vi "TX.vi"() -> ()   [LabVIEW 2014]
uses:
  <vilib>/Analysis/2dsp.llb/Complex FFT.vi
  <instrlib>/niUSRP/niUSRP Fetch Rx Data (CDB).vi
  <vilib>/addons/Modulation/Digital/General/MT Map QAM Symbols to Bits.vi
  <vilib>/Analysis/NI_AALPro.lvlib
  <vilib>/addons/Modulation/niDMT.lvlib
panel:
  in  "PN sequence order (9) 2":i32=9 caption="PN sequence order (9)"
  in  "Frame Instruction 2":T1
  in  "Code Cluster":T2={"Code type"=enum."No code", "Encode factor"=2, "Constraint length(For convolution code)"=3}
  in  "modulation choice 3":T3
  in  "modulation choice 2":T3
  out "Outgoing Constellation":cdb[](graph)=[-0.7071067811865476-0.7071067811865476i, -0.7071067811865476-0.7071067811865476i, -0.7071067811865476-0.7071067811865476i, 0.7071067811865476-0.7071067811865476i, 0.7071067811865476-0.7071067811865476i, 0.7071067811865476+0.7071067811865476i, 0.7071067811865476-0.7071067811865476i, -0.7071067811865476-0.7071067811865476i, 0.7071067811865476+0.7071067811865476i, -0.7071067811865476+0.7071067811865476i, -0.7071067811865476-0.7071067811865476i, -0.7071067811865476+0.7071067811865476i, -0.7071067811865476+0.7071067811865476i, 0.7071067811865476-0.7071067811865476i, -0.7071067811865476+0.7071067811865476i, -0.7071067811865476+0.7071067811865476i, 0.7071067811865476-0.7071067811865476i, -0.7071067811865476+0.7071067811865476i, -0.7071067811865476-0.7071067811865476i, 0.7071067811865476-0.7071067811865476i, 0.7071067811865476+0.7071067811865476i, -0.7071067811865476-0.7071067811865476i, -0.7071067811865476-0.7071067811865476i, 0.7071067811865476-0.7071067811865476i, -0.7071067811865476-0.7071067811865476i, 0.7071067811865476-0.7071067811865476i, 0.7071067811865476-0.7071067811865476i, 0.7071067811865476+0.7071067811865476i, 0.7071067811865476+0.7071067811865476i, -0.7071067811865476-0.7071067811865476i, -0.7071067811865476+0.7071067811865476i, -0.7071067811865476+0.7071067811865476i, 0.7071067811865476-0.7071067811865476i, -0.7071067811865476-0.7071067811865476i, -0.7071067811865476+0.7071067811865476i, -0.7071067811865476-0.7071067811865476i, -0.7071067811865476+0.7071067811865476i, 0.7071067811865476-0.7071067811865476i, 0.7071067811865476+0.7071067811865476i, 0.7071067811865476+0.7071067811865476i, 0.7071067811865476-0.7071067811865476i, -0.7071067811865476-0.7071067811865476i, -0.7071067811865476+0.7071067811865476i, -0.7071067811865476+0.7071067811865476i, -0.7071067811865476-0.7071067811865476i, -0.7071067811865476-0.7071067811865476i, -0.7071067811865476+0.7071067811865476i, -0.7071067811865476+0.7071067811865476i, -0.7071067811865476+0.7071067811865476i, -0.7071067811865476+0.7071067811865476i, 0.7071067811865476+0.7071067811865476i, 0.7071067811865476+0.7071067811865476i, 0.7071067811865476+0.7071067811865476i, 0.7071067811865476-0.7071067811865476i, 0.7071067811865476-0.7071067811865476i, -0.7071067811865476+0.7071067811865476i, -0.7071067811865476+0.7071067811865476i, -0.7071067811865476+0.7071067811865476i, -0.7071067811865476-0.7071067811865476i, 0.7071067811865476-0.7071067811865476i, -0.7071067811865476+0.7071067811865476i, -0.7071067811865476+0.7071067811865476i, -0.7071067811865476-0.7071067811865476i, -0.7071067811865476+0.7071067811865476i, -0.7071067811865476-0.7071067811865476i, 0.7071067811865476+0.7071067811865476i, 0.7071067811865476+0.7071067811865476i, 0.7071067811865476+0.7071067811865476i, -0.7071067811865476-0.7071067811865476i, 0.7071067811865476-0.7071067811865476i, -0.7071067811865476+0.7071067811865476i, -0.7071067811865476-0.7071067811865476i, -0.7071067811865476+0.7071067811865476i, 0.7071067811865476+0.7071067811865476i, 0.7071067811865476-0.7071067811865476i, -0.7071067811865476+0.7071067811865476i, -0.7071067811865476-0.7071067811865476i, 0.7071067811865476-0.7071067811865476i, 0.7071067811865476-0.7071067811865476i, -0.7071067811865476-0.7071067811865476i, 0.7071067811865476-0.7071067811865476i, 0.7071067811865476-0.7071067811865476i, 0.7071067811865476-0.7071067811865476i, 0.7071067811865476+0.7071067811865476i, 0.7071067811865476-0.7071067811865476i, -0.7071067811865476+0.7071067811865476i, 0.7071067811865476+0.7071067811865476i, 0.7071067811865476+0.7071067811865476i, -0.7071067811865476-0.7071067811865476i, 0.7071067811865476+0.7071067811865476i, -0.7071067811865476-0.7071067811865476i, 0.7071067811865476-0.7071067811865476i, 0.7071067811865476+0.7071067811865476i, -0.7071067811865476+0.7071067811865476i, -0.7071067811865476+0.7071067811865476i, -0.7071067811865476-0.7071067811865476i, 0.7071067811865476-0.7071067811865476i, -0.7071067811865476-0.7071067811865476i, -0.7071067811865476+0.7071067811865476i, 0.7071067811865476-0.7071067811865476i, -0.7071067811865476+0.7071067811865476i, 0.7071067811865476-0.7071067811865476i, 0.7071067811865476-0.7071067811865476i, 0.7071067811865476+0.7071067811865476i, -0.7071067811865476+0.7071067811865476i, -0.7071067811865476-0.7071067811865476i, -0.7071067811865476+0.7071067811865476i, -0.7071067811865476-0.7071067811865476i, 0.7071067811865476-0.7071067811865476i, 0.7071067811865476+0.7071067811865476i, -0.7071067811865476+0.7071067811865476i, -0.7071067811865476-0.7071067811865476i, -0.7071067811865476-0.7071067811865476i, -0.7071067811865476-0.7071067811865476i, -0.7071067811865476-0.7071067811865476i, 0.7071067811865476+0.7071067811865476i, 0.7071067811865476+0.7071067811865476i, -0.7071067811865476+0.7071067811865476i, -0.7071067811865476-0.7071067811865476i, 0.7071067811865476-0.7071067811865476i, -0.7071067811865476-0.7071067811865476i, -0.7071067811865476-0.7071067811865476i, 0.7071067811865476-0.7071067811865476i, 0.7071067811865476+0.7071067811865476i, 0.7071067811865476-0.7071067811865476i, -0.7071067811865476-0.7071067811865476i, 0.7071067811865476-0.7071067811865476i, -0.7071067811865476+0.7071067811865476i, 0.7071067811865476-0.7071067811865476i, -0.7071067811865476+0.7071067811865476i, 0.7071067811865476+0.7071067811865476i, 0.7071067811865476+0.7071067811865476i, -0.7071067811865476+0.7071067811865476i, 0.7071067811865476+0.7071067811865476i, 0.7071067811865476-0.7071067811865476i, 0.7071067811865476-0.7071067811865476i, -0.7071067811865476+0.7071067811865476i, -0.7071067811865476-0.7071067811865476i, -0.7071067811865476+0.7071067811865476i, 0.7071067811865476-0.7071067811865476i, 0.7071067811865476-0.7071067811865476i, 0.7071067811865476+0.7071067811865476i, -0.7071067811865476-0.7071067811865476i, -0.7071067811865476-0.7071067811865476i, 0.7071067811865476+0.7071067811865476i, -0.7071067811865476-0.7071067811865476i, -0.7071067811865476-0.7071067811865476i, 0.7071067811865476-0.7071067811865476i, -0.7071067811865476+0.7071067811865476i, 0.7071067811865476-0.7071067811865476i, -0.7071067811865476-0.7071067811865476i, 0.7071067811865476+0.7071067811865476i, -0.7071067811865476+0.7071067811865476i, -0.7071067811865476+0.7071067811865476i, -0.7071067811865476+0.7071067811865476i, 0.7071067811865476+0.7071067811865476i, 0.7071067811865476-0.7071067811865476i, 0.7071067811865476+0.7071067811865476i, -0.7071067811865476-0.7071067811865476i, 0.7071067811865476-0.7071067811865476i, 0.7071067811865476+0.7071067811865476i, -0.7071067811865476-0.7071067811865476i, -0.7071067811865476+0.7071067811865476i, 0.7071067811865476-0.7071067811865476i, 0.7071067811865476-0.7071067811865476i, 0.7071067811865476-0.7071067811865476i, -0.7071067811865476-0.7071067811865476i, 0.7071067811865476-0.7071067811865476i, 0.7071067811865476+0.7071067811865476i, 0.7071067811865476-0.7071067811865476i, -0.7071067811865476+0.7071067811865476i, 0.7071067811865476-0.7071067811865476i, 0.7071067811865476+0.7071067811865476i, 0.7071067811865476-0.7071067811865476i, 0.7071067811865476+0.7071067811865476i, 0.7071067811865476-0.7071067811865476i, 0.7071067811865476+0.7071067811865476i, 0.7071067811865476+0.7071067811865476i, 0.7071067811865476+0.7071067811865476i, -0.7071067811865476+0.7071067811865476i, 0.7071067811865476+0.7071067811865476i, 0.7071067811865476+0.7071067811865476i, 0.7071067811865476-0.7071067811865476i, 0.7071067811865476+0.7071067811865476i, -0.7071067811865476-0.7071067811865476i, 0.7071067811865476+0.7071067811865476i, 0.7071067811865476+0.7071067811865476i, 0.7071067811865476-0.7071067811865476i, -0.7071067811865476+0.7071067811865476i, -0.7071067811865476-0.7071067811865476i, 0.7071067811865476+0.7071067811865476i, 0.7071067811865476-0.7071067811865476i, 0.7071067811865476-0.7071067811865476i, 0.7071067811865476-0.7071067811865476i, -0.7071067811865476-0.7071067811865476i, 0.7071067811865476+0.7071067811865476i, 0.7071067811865476+0.7071067811865476i, -0.7071067811865476-0.7071067811865476i, -0.7071067811865476+0.7071067811865476i, -0.7071067811865476-0.7071067811865476i, 0.7071067811865476-0.7071067811865476i, 0.7071067811865476-0.7071067811865476i, -0.7071067811865476+0.7071067811865476i, 0.7071067811865476-0.7071067811865476i, -0.7071067811865476-0.7071067811865476i, 0.7071067811865476-0.7071067811865476i, -0.7071067811865476+0.7071067811865476i, 0.7071067811865476+0.7071067811865476i, -0.7071067811865476+0.7071067811865476i, -0.7071067811865476+0.7071067811865476i, 0.7071067811865476+0.7071067811865476i, 0.7071067811865476+0.7071067811865476i, 0.7071067811865476-0.7071067811865476i, 0.7071067811865476-0.7071067811865476i, -0.7071067811865476-0.7071067811865476i, -0.7071067811865476+0.7071067811865476i, 0.7071067811865476+0.7071067811865476i, -0.7071067811865476-0.7071067811865476i, -0.7071067811865476-0.7071067811865476i, -0.7071067811865476-0.7071067811865476i, -0.7071067811865476+0.7071067811865476i, 0.7071067811865476-0.7071067811865476i, -0.7071067811865476+0.7071067811865476i, 0.7071067811865476+0.7071067811865476i, 0.7071067811865476-0.7071067811865476i, -0.7071067811865476+0.7071067811865476i, -0.7071067811865476+0.7071067811865476i, 0.7071067811865476-0.7071067811865476i, -0.7071067811865476-0.7071067811865476i, -0.7071067811865476-0.7071067811865476i, -0.7071067811865476-0.7071067811865476i, 0.7071067811865476+0.7071067811865476i, 0.7071067811865476-0.7071067811865476i, -0.7071067811865476+0.7071067811865476i, 0.7071067811865476-0.7071067811865476i, 0.7071067811865476-0.7071067811865476i, 0.7071067811865476-0.7071067811865476i, -0.7071067811865476+0.7071067811865476i, 0.7071067811865476-0.7071067811865476i, -0.7071067811865476+0.7071067811865476i, 0.7071067811865476-0.7071067811865476i, 0.7071067811865476+0.7071067811865476i, 0.7071067811865476+0.7071067811865476i, 0.7071067811865476+0.7071067811865476i, -0.7071067811865476-0.7071067811865476i, 0.7071067811865476+0.7071067811865476i, -0.7071067811865476+0.7071067811865476i, 0.7071067811865476-0.7071067811865476i, -0.7071067811865476+0.7071067811865476i, -0.7071067811865476+0.7071067811865476i, 0.7071067811865476+0.7071067811865476i, -0.7071067811865476+0.7071067811865476i, 0.7071067811865476-0.7071067811865476i, 0.7071067811865476-0.7071067811865476i, -0.7071067811865476+0.7071067811865476i, -0.7071067811865476+0.7071067811865476i, -0.7071067811865476-0.7071067811865476i, -0.7071067811865476-0.7071067811865476i, -0.7071067811865476-0.7071067811865476i, -0.7071067811865476+0.7071067811865476i, 0.7071067811865476+0.7071067811865476i, -0.7071067811865476+0.7071067811865476i, -0.7071067811865476+0.7071067811865476i, 0.7071067811865476-0.7071067811865476i, 0.7071067811865476+0.7071067811865476i, -0.7071067811865476-0.7071067811865476i, 0.7071067811865476-0.7071067811865476i, 0.7071067811865476-0.7071067811865476i, -0.7071067811865476-0.7071067811865476i, 0.7071067811865476+0.7071067811865476i, 0.7071067811865476-0.7071067811865476i, -0.7071067811865476-0.7071067811865476i, 0.7071067811865476+0.7071067811865476i, -0.7071067811865476-0.7071067811865476i, -0.7071067811865476-0.7071067811865476i, 0.7071067811865476+0.7071067811865476i, -0.7071067811865476+0.7071067811865476i, -0.7071067811865476-0.7071067811865476i, -0.7071067811865476-0.7071067811865476i, -0.7071067811865476+0.7071067811865476i, -0.7071067811865476-0.7071067811865476i, -0.7071067811865476+0.7071067811865476i, 0.7071067811865476+0.7071067811865476i, 0.7071067811865476+0.7071067811865476i, -0.7071067811865476+0.7071067811865476i, 0.7071067811865476-0.7071067811865476i, 0.7071067811865476-0.7071067811865476i, -0.7071067811865476-0.7071067811865476i, -0.7071067811865476+0.7071067811865476i, 0.7071067811865476-0.7071067811865476i, -0.7071067811865476-0.7071067811865476i, 0.7071067811865476-0.7071067811865476i, -0.7071067811865476-0.7071067811865476i, 0.7071067811865476+0.7071067811865476i, 0.7071067811865476+0.7071067811865476i, -0.7071067811865476+0.7071067811865476i, -0.7071067811865476+0.7071067811865476i, 0.7071067811865476-0.7071067811865476i, 0.7071067811865476-0.7071067811865476i, -0.7071067811865476-0.7071067811865476i, -0.7071067811865476-0.7071067811865476i, 0.7071067811865476-0.7071067811865476i, 0.7071067811865476-0.7071067811865476i, 0.7071067811865476-0.7071067811865476i, 0.7071067811865476-0.7071067811865476i, 0.7071067811865476-0.7071067811865476i, 0.7071067811865476+0.7071067811865476i, 0.7071067811865476+0.7071067811865476i, -0.7071067811865476+0.7071067811865476i, -0.7071067811865476+0.7071067811865476i, 0.7071067811865476+0.7071067811865476i, 0.7071067811865476-0.7071067811865476i, 0.7071067811865476-0.7071067811865476i, -0.7071067811865476-0.7071067811865476i, -0.7071067811865476-0.7071067811865476i, 0.7071067811865476+0.7071067811865476i, 0.7071067811865476-0.7071067811865476i, -0.7071067811865476-0.7071067811865476i, 0.7071067811865476-0.7071067811865476i, -0.7071067811865476-0.7071067811865476i, 0.7071067811865476-0.7071067811865476i, 0.7071067811865476+0.7071067811865476i, 0.7071067811865476+0.7071067811865476i, -0.7071067811865476+0.7071067811865476i, -0.7071067811865476-0.7071067811865476i, 0.7071067811865476+0.7071067811865476i, -0.7071067811865476-0.7071067811865476i, 0.7071067811865476-0.7071067811865476i, 0.7071067811865476-0.7071067811865476i, -0.7071067811865476+0.7071067811865476i, 0.7071067811865476+0.7071067811865476i, -0.7071067811865476-0.7071067811865476i, -0.7071067811865476-0.7071067811865476i, -0.7071067811865476+0.7071067811865476i, -0.7071067811865476+0.7071067811865476i, -0.7071067811865476-0.7071067811865476i, -0.7071067811865476+0.7071067811865476i, -0.7071067811865476+0.7071067811865476i, 0.7071067811865476+0.7071067811865476i, -0.7071067811865476+0.7071067811865476i, 0.7071067811865476+0.7071067811865476i, 0.7071067811865476-0.7071067811865476i, 0.7071067811865476+0.7071067811865476i, -0.7071067811865476+0.7071067811865476i, 0.7071067811865476-0.7071067811865476i, -0.7071067811865476+0.7071067811865476i, -0.7071067811865476-0.7071067811865476i, 0.7071067811865476+0.7071067811865476i, 0.7071067811865476+0.7071067811865476i, 0.7071067811865476-0.7071067811865476i, -0.7071067811865476-0.7071067811865476i, -0.7071067811865476-0.7071067811865476i, -0.7071067811865476+0.7071067811865476i, 0.7071067811865476-0.7071067811865476i, -0.7071067811865476-0.7071067811865476i, 0.7071067811865476+0.7071067811865476i, -0.7071067811865476-0.7071067811865476i, -0.7071067811865476+0.7071067811865476i, 0.7071067811865476+0.7071067811865476i, 0.7071067811865476+0.7071067811865476i, -0.7071067811865476-0.7071067811865476i, 0.7071067811865476-0.7071067811865476i, -0.7071067811865476-0.7071067811865476i, -0.7071067811865476-0.7071067811865476i, 0.7071067811865476+0.7071067811865476i, 0.7071067811865476+0.7071067811865476i, -0.7071067811865476-0.7071067811865476i, -0.7071067811865476-0.7071067811865476i, -0.7071067811865476-0.7071067811865476i, -0.7071067811865476-0.7071067811865476i, 0.7071067811865476-0.7071067811865476i, 0.7071067811865476+0.7071067811865476i, 0.7071067811865476+0.7071067811865476i, -0.7071067811865476-0.7071067811865476i, -0.7071067811865476-0.7071067811865476i, -0.7071067811865476+0.7071067811865476i, -0.7071067811865476-0.7071067811865476i, -0.7071067811865476-0.7071067811865476i, 0.7071067811865476+0.7071067811865476i, -0.7071067811865476+0.7071067811865476i, -0.7071067811865476+0.7071067811865476i, -0.7071067811865476-0.7071067811865476i, 0.7071067811865476+0.7071067811865476i, -0.7071067811865476-0.7071067811865476i, 0.7071067811865476+0.7071067811865476i, 0.7071067811865476-0.7071067811865476i, 0.7071067811865476+0.7071067811865476i, 0.7071067811865476+0.7071067811865476i, 0.7071067811865476-0.7071067811865476i, -0.7071067811865476+0.7071067811865476i, -0.7071067811865476+0.7071067811865476i, 0.7071067811865476+0.7071067811865476i, -0.7071067811865476-0.7071067811865476i, 0.7071067811865476-0.7071067811865476i, -0.7071067811865476-0.7071067811865476i, -0.7071067811865476+0.7071067811865476i, 0.7071067811865476+0.7071067811865476i, -0.7071067811865476+0.7071067811865476i, -0.7071067811865476-0.7071067811865476i, 0.7071067811865476-0.7071067811865476i, -0.7071067811865476+0.7071067811865476i, -0.7071067811865476-0.7071067811865476i, -0.7071067811865476-0.7071067811865476i, 0.7071067811865476+0.7071067811865476i, -0.7071067811865476-0.7071067811865476i, -0.7071067811865476+0.7071067811865476i, 0.7071067811865476-0.7071067811865476i, 0.7071067811865476+0.7071067811865476i, 0.7071067811865476-0.7071067811865476i, 0.7071067811865476-0.7071067811865476i, 0.7071067811865476-0.7071067811865476i, -0.7071067811865476+0.7071067811865476i, 0.7071067811865476+0.7071067811865476i, -0.7071067811865476+0.7071067811865476i, -0.7071067811865476-0.7071067811865476i, 0.7071067811865476+0.7071067811865476i, -0.7071067811865476+0.7071067811865476i, 0.7071067811865476-0.7071067811865476i, -0.7071067811865476-0.7071067811865476i, -0.7071067811865476+0.7071067811865476i, -0.7071067811865476+0.7071067811865476i, -0.7071067811865476+0.7071067811865476i, -0.7071067811865476-0.7071067811865476i, 0.7071067811865476+0.7071067811865476i, -0.7071067811865476+0.7071067811865476i, 0.7071067811865476+0.7071067811865476i, -0.7071067811865476-0.7071067811865476i, 0.7071067811865476+0.7071067811865476i, -0.7071067811865476+0.7071067811865476i, 0.7071067811865476+0.7071067811865476i, -0.7071067811865476+0.7071067811865476i, 0.7071067811865476+0.7071067811865476i, 0.7071067811865476+0.7071067811865476i, 0.7071067811865476+0.7071067811865476i, 0.7071067811865476+0.7071067811865476i, 0.7071067811865476-0.7071067811865476i, 0.7071067811865476+0.7071067811865476i, -0.7071067811865476+0.7071067811865476i, 0.7071067811865476+0.7071067811865476i, -0.7071067811865476+0.7071067811865476i, 0.7071067811865476-0.7071067811865476i, 0.7071067811865476+0.7071067811865476i, -0.7071067811865476+0.7071067811865476i, 0.7071067811865476+0.7071067811865476i, -0.7071067811865476-0.7071067811865476i, 0.7071067811865476-0.7071067811865476i, -0.7071067811865476+0.7071067811865476i, -0.7071067811865476+0.7071067811865476i, -0.7071067811865476+0.7071067811865476i, -0.7071067811865476+0.7071067811865476i, 0.7071067811865476-0.7071067811865476i, 0.7071067811865476+0.7071067811865476i, -0.7071067811865476+0.7071067811865476i, 0.7071067811865476-0.7071067811865476i, -0.7071067811865476-0.7071067811865476i, -0.7071067811865476-0.7071067811865476i, -0.7071067811865476+0.7071067811865476i, 0.7071067811865476+0.7071067811865476i, -0.7071067811865476-0.7071067811865476i, -0.7071067811865476+0.7071067811865476i, -0.7071067811865476-0.7071067811865476i, 0.7071067811865476+0.7071067811865476i, 0.7071067811865476-0.7071067811865476i, 0.7071067811865476+0.7071067811865476i, 0.7071067811865476-0.7071067811865476i, 0.7071067811865476-0.7071067811865476i, 0.7071067811865476+0.7071067811865476i, -0.7071067811865476+0.7071067811865476i, -0.7071067811865476+0.7071067811865476i, -0.7071067811865476+0.7071067811865476i, 0.7071067811865476-0.7071067811865476i, 0.7071067811865476-0.7071067811865476i, -0.7071067811865476+0.7071067811865476i, -0.7071067811865476-0.7071067811865476i, -0.7071067811865476-0.7071067811865476i, 0.7071067811865476-0.7071067811865476i, -0.7071067811865476-0.7071067811865476i, 0.7071067811865476+0.7071067811865476i, 0.7071067811865476-0.7071067811865476i, -0.7071067811865476+0.7071067811865476i, 0.7071067811865476+0.7071067811865476i, 0.7071067811865476-0.7071067811865476i, -0.7071067811865476-0.7071067811865476i, -0.7071067811865476+0.7071067811865476i, -0.7071067811865476-0.7071067811865476i, -0.7071067811865476-0.7071067811865476i, 0.7071067811865476-0.7071067811865476i, -0.7071067811865476+0.7071067811865476i, 0.7071067811865476+0.7071067811865476i, -0.7071067811865476-0.7071067811865476i, -0.7071067811865476+0.7071067811865476i, -0.7071067811865476+0.7071067811865476i, 0.7071067811865476+0.7071067811865476i, -0.7071067811865476-0.7071067811865476i, 0.7071067811865476+0.7071067811865476i, -0.7071067811865476-0.7071067811865476i, 0.7071067811865476+0.7071067811865476i, 0.7071067811865476+0.7071067811865476i, 0.7071067811865476+0.7071067811865476i, -0.7071067811865476+0.7071067811865476i, 0.7071067811865476-0.7071067811865476i, 0.7071067811865476+0.7071067811865476i, -0.7071067811865476-0.7071067811865476i, 0.7071067811865476+0.7071067811865476i, 0.7071067811865476-0.7071067811865476i, 0.7071067811865476-0.7071067811865476i, 0.7071067811865476+0.7071067811865476i, -0.7071067811865476-0.7071067811865476i, -0.7071067811865476+0.7071067811865476i, 0.7071067811865476+0.7071067811865476i, 0.7071067811865476-0.7071067811865476i, -0.7071067811865476-0.7071067811865476i, -0.7071067811865476-0.7071067811865476i, -0.7071067811865476-0.7071067811865476i, 0.7071067811865476-0.7071067811865476i, 0.7071067811865476-0.7071067811865476i, 0.7071067811865476+0.7071067811865476i, 0.7071067811865476-0.7071067811865476i, -0.7071067811865476-0.7071067811865476i, 0.7071067811865476+0.7071067811865476i, -0.7071067811865476+0.7071067811865476i, -0.7071067811865476-0.7071067811865476i, -0.7071067811865476+0.7071067811865476i, -0.7071067811865476+0.7071067811865476i, 0.7071067811865476-0.7071067811865476i, -0.7071067811865476+0.7071067811865476i, -0.7071067811865476+0.7071067811865476i, 0.7071067811865476-0.7071067811865476i, -0.7071067811865476+0.7071067811865476i, -0.7071067811865476-0.7071067811865476i, 0.7071067811865476-0.7071067811865476i, 0.7071067811865476+0.7071067811865476i, -0.7071067811865476-0.7071067811865476i, -0.7071067811865476-0.7071067811865476i, 0.7071067811865476-0.7071067811865476i, -0.7071067811865476-0.7071067811865476i, 0.7071067811865476-0.7071067811865476i, 0.7071067811865476-0.7071067811865476i, 0.7071067811865476+0.7071067811865476i, 0.7071067811865476+0.7071067811865476i, -0.7071067811865476-0.7071067811865476i, -0.7071067811865476+0.7071067811865476i, -0.7071067811865476+0.7071067811865476i, 0.7071067811865476-0.7071067811865476i, -0.7071067811865476-0.7071067811865476i, -0.7071067811865476+0.7071067811865476i, -0.7071067811865476-0.7071067811865476i, -0.7071067811865476+0.7071067811865476i, 0.7071067811865476-0.7071067811865476i, 0.7071067811865476+0.7071067811865476i, 0.7071067811865476+0.7071067811865476i, 0.7071067811865476-0.7071067811865476i, -0.7071067811865476-0.7071067811865476i, -0.7071067811865476+0.7071067811865476i, -0.7071067811865476+0.7071067811865476i, -0.7071067811865476-0.7071067811865476i, -0.7071067811865476-0.7071067811865476i, -0.7071067811865476+0.7071067811865476i, -0.7071067811865476+0.7071067811865476i, -0.7071067811865476+0.7071067811865476i, -0.7071067811865476+0.7071067811865476i, 0.7071067811865476+0.7071067811865476i, 0.7071067811865476+0.7071067811865476i, 0.7071067811865476+0.7071067811865476i, 0.7071067811865476-0.7071067811865476i, 0.7071067811865476-0.7071067811865476i, -0.7071067811865476+0.7071067811865476i, -0.7071067811865476+0.7071067811865476i, -0.7071067811865476+0.7071067811865476i, -0.7071067811865476-0.7071067811865476i, 0.7071067811865476-0.7071067811865476i, -0.7071067811865476+0.7071067811865476i, -0.7071067811865476+0.7071067811865476i, -0.7071067811865476-0.7071067811865476i, -0.7071067811865476+0.7071067811865476i, -0.7071067811865476-0.7071067811865476i, 0.7071067811865476+0.7071067811865476i, 0.7071067811865476+0.7071067811865476i, 0.7071067811865476+0.7071067811865476i, -0.7071067811865476-0.7071067811865476i, 0.7071067811865476-0.7071067811865476i, -0.7071067811865476+0.7071067811865476i, -0.7071067811865476-0.7071067811865476i, -0.7071067811865476+0.7071067811865476i, 0.7071067811865476+0.7071067811865476i, 0.7071067811865476-0.7071067811865476i, -0.7071067811865476+0.7071067811865476i, -0.7071067811865476-0.7071067811865476i, 0.7071067811865476-0.7071067811865476i, 0.7071067811865476-0.7071067811865476i, -0.7071067811865476-0.7071067811865476i, 0.7071067811865476-0.7071067811865476i, 0.7071067811865476-0.7071067811865476i, 0.7071067811865476-0.7071067811865476i, 0.7071067811865476+0.7071067811865476i, 0.7071067811865476-0.7071067811865476i, -0.7071067811865476+0.7071067811865476i, 0.7071067811865476+0.7071067811865476i, 0.7071067811865476+0.7071067811865476i, -0.7071067811865476-0.7071067811865476i, 0.7071067811865476+0.7071067811865476i, -0.7071067811865476-0.7071067811865476i, 0.7071067811865476-0.7071067811865476i, 0.7071067811865476+0.7071067811865476i, -0.7071067811865476+0.7071067811865476i, -0.7071067811865476+0.7071067811865476i, -0.7071067811865476-0.7071067811865476i, 0.7071067811865476-0.7071067811865476i, -0.7071067811865476-0.7071067811865476i, -0.7071067811865476+0.7071067811865476i, 0.7071067811865476-0.7071067811865476i, -0.7071067811865476+0.7071067811865476i, 0.7071067811865476-0.7071067811865476i, 0.7071067811865476-0.7071067811865476i, 0.7071067811865476+0.7071067811865476i, -0.7071067811865476+0.7071067811865476i, -0.7071067811865476-0.7071067811865476i, -0.7071067811865476+0.7071067811865476i, -0.7071067811865476-0.7071067811865476i, 0.7071067811865476-0.7071067811865476i, 0.7071067811865476+0.7071067811865476i, -0.7071067811865476+0.7071067811865476i, -0.7071067811865476-0.7071067811865476i, -0.7071067811865476-0.7071067811865476i, -0.7071067811865476-0.7071067811865476i, -0.7071067811865476-0.7071067811865476i, 0.7071067811865476+0.7071067811865476i, 0.7071067811865476+0.7071067811865476i, -0.7071067811865476+0.7071067811865476i, -0.7071067811865476-0.7071067811865476i, 0.7071067811865476-0.7071067811865476i, -0.7071067811865476-0.7071067811865476i, -0.7071067811865476-0.7071067811865476i, 0.7071067811865476-0.7071067811865476i, 0.7071067811865476+0.7071067811865476i, 0.7071067811865476-0.7071067811865476i, -0.7071067811865476-0.7071067811865476i, 0.7071067811865476-0.7071067811865476i, -0.7071067811865476+0.7071067811865476i, 0.7071067811865476-0.7071067811865476i, -0.7071067811865476+0.7071067811865476i, 0.7071067811865476+0.7071067811865476i, 0.7071067811865476+0.7071067811865476i, -0.7071067811865476+0.7071067811865476i, 0.7071067811865476+0.7071067811865476i, 0.7071067811865476-0.7071067811865476i, 0.7071067811865476-0.7071067811865476i, -0.7071067811865476+0.7071067811865476i, -0.7071067811865476-0.7071067811865476i, -0.7071067811865476+0.7071067811865476i, 0.7071067811865476-0.7071067811865476i, 0.7071067811865476-0.7071067811865476i, 0.7071067811865476+0.7071067811865476i, -0.7071067811865476-0.7071067811865476i, -0.7071067811865476-0.7071067811865476i, 0.7071067811865476+0.7071067811865476i, -0.7071067811865476-0.7071067811865476i, -0.7071067811865476-0.7071067811865476i, 0.7071067811865476-0.7071067811865476i, -0.7071067811865476+0.7071067811865476i, 0.7071067811865476-0.7071067811865476i, -0.7071067811865476-0.7071067811865476i, 0.7071067811865476+0.7071067811865476i, -0.7071067811865476+0.7071067811865476i, -0.7071067811865476+0.7071067811865476i, -0.7071067811865476+0.7071067811865476i, 0.7071067811865476+0.7071067811865476i, 0.7071067811865476-0.7071067811865476i, 0.7071067811865476+0.7071067811865476i, -0.7071067811865476-0.7071067811865476i, 0.7071067811865476-0.7071067811865476i, 0.7071067811865476+0.7071067811865476i, -0.7071067811865476-0.7071067811865476i, -0.7071067811865476+0.7071067811865476i, 0.7071067811865476-0.7071067811865476i, 0.7071067811865476-0.7071067811865476i, 0.7071067811865476-0.7071067811865476i, -0.7071067811865476-0.7071067811865476i, 0.7071067811865476-0.7071067811865476i, 0.7071067811865476+0.7071067811865476i, 0.7071067811865476-0.7071067811865476i, -0.7071067811865476+0.7071067811865476i, 0.7071067811865476-0.7071067811865476i, 0.7071067811865476+0.7071067811865476i, 0.7071067811865476-0.7071067811865476i, 0.7071067811865476+0.7071067811865476i, 0.7071067811865476-0.7071067811865476i, 0.7071067811865476+0.7071067811865476i, 0.7071067811865476+0.7071067811865476i, 0.7071067811865476+0.7071067811865476i, -0.7071067811865476+0.7071067811865476i, 0.7071067811865476+0.7071067811865476i, 0.7071067811865476+0.7071067811865476i, 0.7071067811865476-0.7071067811865476i, 0.7071067811865476+0.7071067811865476i, -0.7071067811865476-0.7071067811865476i, 0.7071067811865476+0.7071067811865476i, 0.7071067811865476+0.7071067811865476i, 0.7071067811865476-0.7071067811865476i, -0.7071067811865476+0.7071067811865476i, -0.7071067811865476-0.7071067811865476i, 0.7071067811865476+0.7071067811865476i, 0.7071067811865476-0.7071067811865476i, 0.7071067811865476-0.7071067811865476i, 0.7071067811865476-0.7071067811865476i, -0.7071067811865476-0.7071067811865476i, 0.7071067811865476+0.7071067811865476i, 0.7071067811865476+0.7071067811865476i, -0.7071067811865476-0.7071067811865476i, -0.7071067811865476+0.7071067811865476i, -0.7071067811865476-0.7071067811865476i, 0.7071067811865476-0.7071067811865476i, 0.7071067811865476-0.7071067811865476i, -0.7071067811865476+0.7071067811865476i, 0.7071067811865476-0.7071067811865476i, -0.7071067811865476-0.7071067811865476i, 0.7071067811865476-0.7071067811865476i, -0.7071067811865476+0.7071067811865476i, 0.7071067811865476+0.7071067811865476i, -0.7071067811865476+0.7071067811865476i, -0.7071067811865476+0.7071067811865476i, 0.7071067811865476+0.7071067811865476i, 0.7071067811865476+0.7071067811865476i, 0.7071067811865476-0.7071067811865476i, 0.7071067811865476-0.7071067811865476i, -0.7071067811865476-0.7071067811865476i, -0.7071067811865476+0.7071067811865476i, 0.7071067811865476+0.7071067811865476i, -0.7071067811865476-0.7071067811865476i, -0.7071067811865476-0.7071067811865476i, -0.7071067811865476-0.7071067811865476i, -0.7071067811865476+0.7071067811865476i, 0.7071067811865476-0.7071067811865476i, -0.7071067811865476+0.7071067811865476i, 0.7071067811865476+0.7071067811865476i, 0.7071067811865476-0.7071067811865476i, -0.7071067811865476+0.7071067811865476i, -0.7071067811865476+0.7071067811865476i, 0.7071067811865476-0.7071067811865476i, -0.7071067811865476-0.7071067811865476i, -0.7071067811865476-0.7071067811865476i, -0.7071067811865476-0.7071067811865476i, 0.7071067811865476+0.7071067811865476i, 0.7071067811865476-0.7071067811865476i, -0.7071067811865476+0.7071067811865476i, 0.7071067811865476-0.7071067811865476i, 0.7071067811865476-0.7071067811865476i, 0.7071067811865476-0.7071067811865476i, -0.7071067811865476+0.7071067811865476i, 0.7071067811865476-0.7071067811865476i, -0.7071067811865476+0.7071067811865476i, 0.7071067811865476-0.7071067811865476i, 0.7071067811865476+0.7071067811865476i, 0.7071067811865476+0.7071067811865476i, 0.7071067811865476+0.7071067811865476i, -0.7071067811865476-0.7071067811865476i, 0.7071067811865476+0.7071067811865476i, -0.7071067811865476+0.7071067811865476i, 0.7071067811865476-0.7071067811865476i, -0.7071067811865476+0.7071067811865476i, -0.7071067811865476+0.7071067811865476i, 0.7071067811865476+0.7071067811865476i, -0.7071067811865476+0.7071067811865476i, 0.7071067811865476-0.7071067811865476i, 0.7071067811865476-0.7071067811865476i, -0.7071067811865476+0.7071067811865476i, -0.7071067811865476+0.7071067811865476i, -0.7071067811865476-0.7071067811865476i, -0.7071067811865476-0.7071067811865476i, -0.7071067811865476-0.7071067811865476i, -0.7071067811865476+0.7071067811865476i, 0.7071067811865476+0.7071067811865476i, -0.7071067811865476+0.7071067811865476i, -0.7071067811865476+0.7071067811865476i, 0.7071067811865476-0.7071067811865476i, 0.7071067811865476+0.7071067811865476i, -0.7071067811865476-0.7071067811865476i, 0.7071067811865476-0.7071067811865476i, 0.7071067811865476-0.7071067811865476i, -0.7071067811865476-0.7071067811865476i, 0.7071067811865476+0.7071067811865476i, 0.7071067811865476-0.7071067811865476i, -0.7071067811865476-0.7071067811865476i, 0.7071067811865476+0.7071067811865476i, -0.7071067811865476-0.7071067811865476i, -0.7071067811865476-0.7071067811865476i, 0.7071067811865476+0.7071067811865476i, -0.7071067811865476+0.7071067811865476i, -0.7071067811865476-0.7071067811865476i, -0.7071067811865476-0.7071067811865476i, -0.7071067811865476+0.7071067811865476i, -0.7071067811865476-0.7071067811865476i, -0.7071067811865476+0.7071067811865476i, 0.7071067811865476+0.7071067811865476i, 0.7071067811865476+0.7071067811865476i, -0.7071067811865476+0.7071067811865476i, 0.7071067811865476-0.7071067811865476i, 0.7071067811865476-0.7071067811865476i, -0.7071067811865476-0.7071067811865476i, -0.7071067811865476+0.7071067811865476i, 0.7071067811865476-0.7071067811865476i, -0.7071067811865476-0.7071067811865476i, 0.7071067811865476-0.7071067811865476i, -0.7071067811865476-0.7071067811865476i, 0.7071067811865476+0.7071067811865476i, 0.7071067811865476+0.7071067811865476i, -0.7071067811865476+0.7071067811865476i, -0.7071067811865476+0.7071067811865476i, 0.7071067811865476-0.7071067811865476i, 0.7071067811865476-0.7071067811865476i, -0.7071067811865476-0.7071067811865476i, -0.7071067811865476-0.7071067811865476i, 0.7071067811865476-0.7071067811865476i, 0.7071067811865476-0.7071067811865476i, 0.7071067811865476-0.7071067811865476i, 0.7071067811865476-0.7071067811865476i, 0.7071067811865476-0.7071067811865476i, 0.7071067811865476+0.7071067811865476i, 0.7071067811865476+0.7071067811865476i, -0.7071067811865476+0.7071067811865476i, -0.7071067811865476+0.7071067811865476i, 0.7071067811865476+0.7071067811865476i, 0.7071067811865476-0.7071067811865476i, 0.7071067811865476-0.7071067811865476i, -0.7071067811865476-0.7071067811865476i, -0.7071067811865476-0.7071067811865476i, 0.7071067811865476+0.7071067811865476i, 0.7071067811865476-0.7071067811865476i, -0.7071067811865476-0.7071067811865476i, 0.7071067811865476-0.7071067811865476i, -0.7071067811865476-0.7071067811865476i, 0.7071067811865476-0.7071067811865476i, 0.7071067811865476+0.7071067811865476i, 0.7071067811865476+0.7071067811865476i, -0.7071067811865476+0.7071067811865476i, -0.7071067811865476-0.7071067811865476i, 0.7071067811865476+0.7071067811865476i, -0.7071067811865476-0.7071067811865476i, 0.7071067811865476-0.7071067811865476i, 0.7071067811865476-0.7071067811865476i, -0.7071067811865476+0.7071067811865476i, 0.7071067811865476+0.7071067811865476i, -0.7071067811865476-0.7071067811865476i, -0.7071067811865476-0.7071067811865476i, -0.7071067811865476+0.7071067811865476i, -0.7071067811865476+0.7071067811865476i, -0.7071067811865476-0.7071067811865476i, -0.7071067811865476+0.7071067811865476i, -0.7071067811865476+0.7071067811865476i, 0.7071067811865476+0.7071067811865476i, -0.7071067811865476+0.7071067811865476i, 0.7071067811865476+0.7071067811865476i, 0.7071067811865476-0.7071067811865476i, 0.7071067811865476+0.7071067811865476i, -0.7071067811865476+0.7071067811865476i, 0.7071067811865476-0.7071067811865476i, -0.7071067811865476+0.7071067811865476i, -0.7071067811865476-0.7071067811865476i, 0.7071067811865476+0.7071067811865476i, 0.7071067811865476+0.7071067811865476i, 0.7071067811865476-0.7071067811865476i, -0.7071067811865476-0.7071067811865476i, -0.7071067811865476-0.7071067811865476i, -0.7071067811865476+0.7071067811865476i, 0.7071067811865476-0.7071067811865476i, -0.7071067811865476-0.7071067811865476i, 0.7071067811865476+0.7071067811865476i, -0.7071067811865476-0.7071067811865476i, -0.7071067811865476+0.7071067811865476i, 0.7071067811865476+0.7071067811865476i, 0.7071067811865476+0.7071067811865476i, -0.7071067811865476-0.7071067811865476i, 0.7071067811865476-0.7071067811865476i, -0.7071067811865476-0.7071067811865476i, -0.7071067811865476-0.7071067811865476i, 0.7071067811865476+0.7071067811865476i, 0.7071067811865476+0.7071067811865476i, -0.7071067811865476-0.7071067811865476i, -0.7071067811865476-0.7071067811865476i, -0.7071067811865476-0.7071067811865476i, -0.7071067811865476-0.7071067811865476i, 0.7071067811865476-0.7071067811865476i, 0.7071067811865476+0.7071067811865476i, 0.7071067811865476+0.7071067811865476i, -0.7071067811865476-0.7071067811865476i, -0.7071067811865476-0.7071067811865476i, -0.7071067811865476+0.7071067811865476i, -0.7071067811865476-0.7071067811865476i, -0.7071067811865476-0.7071067811865476i, 0.7071067811865476+0.7071067811865476i, -0.7071067811865476+0.7071067811865476i, -0.7071067811865476+0.7071067811865476i, -0.7071067811865476-0.7071067811865476i, 0.7071067811865476+0.7071067811865476i, -0.7071067811865476-0.7071067811865476i, 0.7071067811865476+0.7071067811865476i, 0.7071067811865476-0.7071067811865476i, 0.7071067811865476+0.7071067811865476i, 0.7071067811865476+0.7071067811865476i, 0.7071067811865476-0.7071067811865476i, -0.7071067811865476+0.7071067811865476i, -0.7071067811865476+0.7071067811865476i, 0.7071067811865476+0.7071067811865476i, -0.7071067811865476-0.7071067811865476i, 0.7071067811865476-0.7071067811865476i, -0.7071067811865476-0.7071067811865476i, -0.7071067811865476+0.7071067811865476i, 0.7071067811865476+0.7071067811865476i, -0.7071067811865476+0.7071067811865476i, -0.7071067811865476-0.7071067811865476i, 0.7071067811865476-0.7071067811865476i, -0.7071067811865476+0.7071067811865476i, -0.7071067811865476-0.7071067811865476i, -0.7071067811865476-0.7071067811865476i, 0.7071067811865476+0.7071067811865476i, -0.7071067811865476-0.7071067811865476i, -0.7071067811865476+0.7071067811865476i, 0.7071067811865476-0.7071067811865476i, 0.7071067811865476+0.7071067811865476i, 0.7071067811865476-0.7071067811865476i, 0.7071067811865476-0.7071067811865476i, 0.7071067811865476-0.7071067811865476i, -0.7071067811865476+0.7071067811865476i, 0.7071067811865476+0.7071067811865476i, -0.7071067811865476+0.7071067811865476i, -0.7071067811865476-0.7071067811865476i, 0.7071067811865476+0.7071067811865476i, -0.7071067811865476+0.7071067811865476i, 0.7071067811865476-0.7071067811865476i, -0.7071067811865476-0.7071067811865476i, -0.7071067811865476+0.7071067811865476i, -0.7071067811865476+0.7071067811865476i, -0.7071067811865476+0.7071067811865476i, -0.7071067811865476-0.7071067811865476i, 0.7071067811865476+0.7071067811865476i, -0.7071067811865476+0.7071067811865476i, 0.7071067811865476+0.7071067811865476i, -0.7071067811865476-0.7071067811865476i, 0.7071067811865476+0.7071067811865476i, -0.7071067811865476+0.7071067811865476i, 0.7071067811865476+0.7071067811865476i, -0.7071067811865476+0.7071067811865476i, 0.7071067811865476+0.7071067811865476i, 0.7071067811865476+0.7071067811865476i, 0.7071067811865476+0.7071067811865476i, 0.7071067811865476+0.7071067811865476i, 0.7071067811865476-0.7071067811865476i, 0.7071067811865476+0.7071067811865476i, -0.7071067811865476+0.7071067811865476i, 0.7071067811865476+0.7071067811865476i, -0.7071067811865476+0.7071067811865476i, 0.7071067811865476-0.7071067811865476i, 0.7071067811865476+0.7071067811865476i, -0.7071067811865476+0.7071067811865476i, 0.7071067811865476+0.7071067811865476i, -0.7071067811865476-0.7071067811865476i, 0.7071067811865476-0.7071067811865476i, -0.7071067811865476+0.7071067811865476i, -0.7071067811865476+0.7071067811865476i, -0.7071067811865476+0.7071067811865476i, -0.7071067811865476+0.7071067811865476i, 0.7071067811865476-0.7071067811865476i, 0.7071067811865476+0.7071067811865476i, -0.7071067811865476+0.7071067811865476i, 0.7071067811865476-0.7071067811865476i, -0.7071067811865476-0.7071067811865476i, -0.7071067811865476-0.7071067811865476i, -0.7071067811865476+0.7071067811865476i, 0.7071067811865476+0.7071067811865476i, -0.7071067811865476-0.7071067811865476i, -0.7071067811865476+0.7071067811865476i, -0.7071067811865476-0.7071067811865476i, 0.7071067811865476+0.7071067811865476i, 0.7071067811865476-0.7071067811865476i, 0.7071067811865476+0.7071067811865476i, 0.7071067811865476-0.7071067811865476i, 0.7071067811865476-0.7071067811865476i, 0.7071067811865476+0.7071067811865476i, -0.7071067811865476+0.7071067811865476i, -0.7071067811865476+0.7071067811865476i, -0.7071067811865476+0.7071067811865476i, 0.7071067811865476-0.7071067811865476i, 0.7071067811865476-0.7071067811865476i, -0.7071067811865476+0.7071067811865476i, -0.7071067811865476-0.7071067811865476i, -0.7071067811865476-0.7071067811865476i, 0.7071067811865476-0.7071067811865476i, -0.7071067811865476-0.7071067811865476i, 0.7071067811865476+0.7071067811865476i, 0.7071067811865476-0.7071067811865476i, -0.7071067811865476+0.7071067811865476i, 0.7071067811865476+0.7071067811865476i, 0.7071067811865476-0.7071067811865476i, -0.7071067811865476-0.7071067811865476i, -0.7071067811865476+0.7071067811865476i, -0.7071067811865476-0.7071067811865476i, -0.7071067811865476-0.7071067811865476i, 0.7071067811865476-0.7071067811865476i, -0.7071067811865476+0.7071067811865476i, 0.7071067811865476+0.7071067811865476i, -0.7071067811865476-0.7071067811865476i, -0.7071067811865476+0.7071067811865476i, -0.7071067811865476+0.7071067811865476i, 0.7071067811865476+0.7071067811865476i, -0.7071067811865476-0.7071067811865476i, 0.7071067811865476+0.7071067811865476i, -0.7071067811865476-0.7071067811865476i, 0.7071067811865476+0.7071067811865476i, 0.7071067811865476+0.7071067811865476i, 0.7071067811865476+0.7071067811865476i, -0.7071067811865476+0.7071067811865476i, 0.7071067811865476-0.7071067811865476i, 0.7071067811865476+0.7071067811865476i, -0.7071067811865476-0.7071067811865476i, 0.7071067811865476+0.7071067811865476i, 0.7071067811865476-0.7071067811865476i, 0.7071067811865476-0.7071067811865476i, 0.7071067811865476+0.7071067811865476i, -0.7071067811865476-0.7071067811865476i, -0.7071067811865476+0.7071067811865476i, 0.7071067811865476+0.7071067811865476i, 0.7071067811865476-0.7071067811865476i, -0.7071067811865476-0.7071067811865476i, -0.7071067811865476-0.7071067811865476i, -0.7071067811865476-0.7071067811865476i, 0.7071067811865476-0.7071067811865476i, 0.7071067811865476-0.7071067811865476i, 0.7071067811865476+0.7071067811865476i, 0.7071067811865476-0.7071067811865476i, -0.7071067811865476-0.7071067811865476i, 0.7071067811865476+0.7071067811865476i, -0.7071067811865476+0.7071067811865476i, -0.7071067811865476-0.7071067811865476i, -0.7071067811865476+0.7071067811865476i, -0.7071067811865476+0.7071067811865476i, 0.7071067811865476-0.7071067811865476i, -0.7071067811865476+0.7071067811865476i, -0.7071067811865476+0.7071067811865476i, 0.7071067811865476-0.7071067811865476i, -0.7071067811865476+0.7071067811865476i, -0.7071067811865476-0.7071067811865476i, 0.7071067811865476-0.7071067811865476i, 0.7071067811865476+0.7071067811865476i, -0.7071067811865476-0.7071067811865476i, -0.7071067811865476-0.7071067811865476i, 0.7071067811865476-0.7071067811865476i, -0.7071067811865476-0.7071067811865476i, 0.7071067811865476-0.7071067811865476i, 0.7071067811865476-0.7071067811865476i, 0.7071067811865476+0.7071067811865476i, 0.7071067811865476+0.7071067811865476i, -0.7071067811865476-0.7071067811865476i, -0.7071067811865476+0.7071067811865476i, -0.7071067811865476+0.7071067811865476i, 0.7071067811865476-0.7071067811865476i, -0.7071067811865476-0.7071067811865476i, -0.7071067811865476+0.7071067811865476i, -0.7071067811865476-0.7071067811865476i, -0.7071067811865476+0.7071067811865476i, 0.7071067811865476-0.7071067811865476i, 0.7071067811865476+0.7071067811865476i, 0.7071067811865476+0.7071067811865476i, 0.7071067811865476-0.7071067811865476i, -0.7071067811865476-0.7071067811865476i, -0.7071067811865476+0.7071067811865476i, -0.7071067811865476+0.7071067811865476i, -0.7071067811865476-0.7071067811865476i, -0.7071067811865476-0.7071067811865476i, -0.7071067811865476+0.7071067811865476i, -0.7071067811865476+0.7071067811865476i, -0.7071067811865476+0.7071067811865476i, -0.7071067811865476+0.7071067811865476i, 0.7071067811865476+0.7071067811865476i, 0.7071067811865476+0.7071067811865476i, 0.7071067811865476+0.7071067811865476i, 0.7071067811865476-0.7071067811865476i, 0.7071067811865476-0.7071067811865476i, -0.7071067811865476+0.7071067811865476i, -0.7071067811865476+0.7071067811865476i, -0.7071067811865476+0.7071067811865476i, -0.7071067811865476-0.7071067811865476i, 0.7071067811865476-0.7071067811865476i, -0.7071067811865476+0.7071067811865476i, -0.7071067811865476+0.7071067811865476i, -0.7071067811865476-0.7071067811865476i, -0.7071067811865476+0.7071067811865476i, -0.7071067811865476-0.7071067811865476i, 0.7071067811865476+0.7071067811865476i, 0.7071067811865476+0.7071067811865476i, 0.7071067811865476+0.7071067811865476i, -0.7071067811865476-0.7071067811865476i, 0.7071067811865476-0.7071067811865476i, -0.7071067811865476+0.7071067811865476i, -0.7071067811865476-0.7071067811865476i, -0.7071067811865476+0.7071067811865476i, 0.7071067811865476+0.7071067811865476i, 0.7071067811865476-0.7071067811865476i, -0.7071067811865476+0.7071067811865476i, -0.7071067811865476-0.7071067811865476i, 0.7071067811865476-0.7071067811865476i, 0.7071067811865476-0.7071067811865476i, -0.7071067811865476-0.7071067811865476i, 0.7071067811865476-0.7071067811865476i, 0.7071067811865476-0.7071067811865476i, 0.7071067811865476-0.7071067811865476i, 0.7071067811865476+0.7071067811865476i, 0.7071067811865476-0.7071067811865476i, -0.7071067811865476+0.7071067811865476i, 0.7071067811865476+0.7071067811865476i, 0.7071067811865476+0.7071067811865476i, -0.7071067811865476-0.7071067811865476i, 0.7071067811865476+0.7071067811865476i, -0.7071067811865476-0.7071067811865476i, 0.7071067811865476-0.7071067811865476i, 0.7071067811865476+0.7071067811865476i, -0.7071067811865476+0.7071067811865476i, -0.7071067811865476+0.7071067811865476i, -0.7071067811865476-0.7071067811865476i, 0.7071067811865476-0.7071067811865476i, -0.7071067811865476-0.7071067811865476i, -0.7071067811865476+0.7071067811865476i, 0.7071067811865476-0.7071067811865476i, -0.7071067811865476+0.7071067811865476i, 0.7071067811865476-0.7071067811865476i, 0.7071067811865476-0.7071067811865476i, 0.7071067811865476+0.7071067811865476i, -0.7071067811865476+0.7071067811865476i, -0.7071067811865476-0.7071067811865476i, -0.7071067811865476+0.7071067811865476i, -0.7071067811865476-0.7071067811865476i, 0.7071067811865476-0.7071067811865476i, 0.7071067811865476+0.7071067811865476i, -0.7071067811865476+0.7071067811865476i, -0.7071067811865476-0.7071067811865476i, -0.7071067811865476-0.7071067811865476i, -0.7071067811865476-0.7071067811865476i, -0.7071067811865476-0.7071067811865476i, 0.7071067811865476+0.7071067811865476i, 0.7071067811865476+0.7071067811865476i, -0.7071067811865476+0.7071067811865476i, -0.7071067811865476-0.7071067811865476i, 0.7071067811865476-0.7071067811865476i, -0.7071067811865476-0.7071067811865476i, -0.7071067811865476-0.7071067811865476i, 0.7071067811865476-0.7071067811865476i, 0.7071067811865476+0.7071067811865476i, 0.7071067811865476-0.7071067811865476i, -0.7071067811865476-0.7071067811865476i, 0.7071067811865476-0.7071067811865476i, -0.7071067811865476+0.7071067811865476i, 0.7071067811865476-0.7071067811865476i, -0.7071067811865476+0.7071067811865476i, 0.7071067811865476+0.7071067811865476i, 0.7071067811865476+0.7071067811865476i, -0.7071067811865476+0.7071067811865476i, 0.7071067811865476+0.7071067811865476i, 0.7071067811865476-0.7071067811865476i, 0.7071067811865476-0.7071067811865476i, -0.7071067811865476+0.7071067811865476i, -0.7071067811865476-0.7071067811865476i, -0.7071067811865476+0.7071067811865476i, 0.7071067811865476-0.7071067811865476i, 0.7071067811865476-0.7071067811865476i, 0.7071067811865476+0.7071067811865476i, -0.7071067811865476-0.7071067811865476i, -0.7071067811865476-0.7071067811865476i, 0.7071067811865476+0.7071067811865476i, -0.7071067811865476-0.7071067811865476i, -0.7071067811865476-0.7071067811865476i, 0.7071067811865476-0.7071067811865476i, -0.7071067811865476+0.7071067811865476i, 0.7071067811865476-0.7071067811865476i, -0.7071067811865476-0.7071067811865476i, 0.7071067811865476+0.7071067811865476i, -0.7071067811865476+0.7071067811865476i, -0.7071067811865476+0.7071067811865476i, -0.7071067811865476+0.7071067811865476i, 0.7071067811865476+0.7071067811865476i, 0.7071067811865476-0.7071067811865476i, 0.7071067811865476+0.7071067811865476i, -0.7071067811865476-0.7071067811865476i, 0.7071067811865476-0.7071067811865476i, 0.7071067811865476+0.7071067811865476i, -0.7071067811865476-0.7071067811865476i, -0.7071067811865476+0.7071067811865476i, 0.7071067811865476-0.7071067811865476i, 0.7071067811865476-0.7071067811865476i, 0.7071067811865476-0.7071067811865476i, -0.7071067811865476-0.7071067811865476i, 0.7071067811865476-0.7071067811865476i, 0.7071067811865476+0.7071067811865476i, 0.7071067811865476-0.7071067811865476i, -0.7071067811865476+0.7071067811865476i, 0.7071067811865476-0.7071067811865476i, 0.7071067811865476+0.7071067811865476i, 0.7071067811865476-0.7071067811865476i, 0.7071067811865476+0.7071067811865476i, 0.7071067811865476-0.7071067811865476i, 0.7071067811865476+0.7071067811865476i, 0.7071067811865476+0.7071067811865476i, 0.7071067811865476+0.7071067811865476i, -0.7071067811865476+0.7071067811865476i, 0.7071067811865476+0.7071067811865476i, 0.7071067811865476+0.7071067811865476i, 0.7071067811865476-0.7071067811865476i, 0.7071067811865476+0.7071067811865476i, -0.7071067811865476-0.7071067811865476i, 0.7071067811865476+0.7071067811865476i, 0.7071067811865476+0.7071067811865476i, 0.7071067811865476-0.7071067811865476i, -0.7071067811865476+0.7071067811865476i, -0.7071067811865476-0.7071067811865476i, 0.7071067811865476+0.7071067811865476i, 0.7071067811865476-0.7071067811865476i, 0.7071067811865476-0.7071067811865476i, 0.7071067811865476-0.7071067811865476i, -0.7071067811865476-0.7071067811865476i, 0.7071067811865476+0.7071067811865476i, 0.7071067811865476+0.7071067811865476i, -0.7071067811865476-0.7071067811865476i, -0.7071067811865476+0.7071067811865476i, -0.7071067811865476-0.7071067811865476i, 0.7071067811865476-0.7071067811865476i, 0.7071067811865476-0.7071067811865476i, -0.7071067811865476+0.7071067811865476i, 0.7071067811865476-0.7071067811865476i, -0.7071067811865476-0.7071067811865476i, 0.7071067811865476-0.7071067811865476i, -0.7071067811865476+0.7071067811865476i, 0.7071067811865476+0.7071067811865476i, -0.7071067811865476+0.7071067811865476i, -0.7071067811865476+0.7071067811865476i, 0.7071067811865476+0.7071067811865476i, 0.7071067811865476+0.7071067811865476i, 0.7071067811865476-0.7071067811865476i, 0.7071067811865476-0.7071067811865476i, -0.7071067811865476-0.7071067811865476i, -0.7071067811865476+0.7071067811865476i, 0.7071067811865476+0.7071067811865476i, -0.7071067811865476-0.7071067811865476i, -0.7071067811865476-0.7071067811865476i, -0.7071067811865476-0.7071067811865476i, -0.7071067811865476+0.7071067811865476i, 0.7071067811865476-0.7071067811865476i, -0.7071067811865476+0.7071067811865476i, 0.7071067811865476+0.7071067811865476i, 0.7071067811865476-0.7071067811865476i, -0.7071067811865476+0.7071067811865476i, -0.7071067811865476+0.7071067811865476i, 0.7071067811865476-0.7071067811865476i]
  out "Frame number":dbl
  in  "Tab Control 2":enum32{"Parameters", "Debug", "CFO"}(tab)
  in  "Device names":refnum<k15>="192.168.1.5"
  in  "Active antenna":string="RX1"
  in  "Gain":dbl=10.0 format="%#_6f"
  in  "Carrier frequency":dbl=2450000000.0 format="%#_6p"
  in  "IQ rate 2":dbl=200000.0 format="%#_6p"
  in  "Number of samples":i64=1600
  out "Coerced IQ rate":dbl=100000.0 format="%#_6p"
  in  "stop 2":bool
  out "Output bit stream":i8[](array[numeric]) caption="output bit stream"
  out "error out 2":errorcluster
  out "error out 3":errorcluster
  out "CFOest (Hz)":dbl[](array[numeric])
  out "Magnitude":dbl[](graph)
  out "Phase":dbl[](graph)
  out "FFT {X}":dbl[](graph)
  out "theta":dbl[](graph)
  out "Unequalized Data":cdb[](graph)
  out "Equalized Data":cdb[](graph)
  out "output bit stream":i8[](array[numeric])
  in  "Frame Instruction":T4={"Guard bits"=182.0, "Sync Bits"=20.0, "Message Data"=48.0}
  in  "PN sequence order (9)":i32=9
  in  "Match filtering":bool
  in  "簇":T5={"RX oversample factor"=10, "簇"={"modulation type"=2, "pulse shaping filter"=2, "filter parameters"=0.5, "filter length"=8}} {"簇"."pulse shaping filter" items=["none", "Raised Cosine", "Root Raised Cos", "Gsussian"]; "簇"."modulation type" items=["FSK", "PSK", "QAM", "MSK", "PAM", "ASK"]}
  out "number":u32
  out "number 2":u32
  in  "modulation choice":T3
  in  "Packet Instruction 3":T6={"Code Rates"=4.0, "Length"=12.0, "Destination address"=8.0, "User"=2.0, "Source address "=8.0, " Frame number"=8.0, " Check sum"=16.0}
  in  "Message Text":string="Two roads diverged in a yellow wood,\nAnd sorry I could not travel both\nAnd be one traveler, long I stood\nAnd looked down one as far as I could\nTo where it bent in the undergrowth.\n\nThen took the other, as just as fair,\nAnd having perhaps the better claim,\nBecause it was grassy and wanted wear;\nThough as for that the passing there\nHad worn them really about the same.\n\nAnd both that morning equally lay\nIn leaves no step had trodden black.\nOh, I kept the first for another day!\nYet knowing how way leads on to way,\nI doubted if I should ever come back.\n\nI shall be telling this with a sigh\nSomewhere ages and ages hence:\nTwo roads diverged in a wood, and I--\nI took the one less traveled by,\nAnd that has made all the difference.\n"
  out "Numeric":dbl
  in  "Tab Control":enum32{"Parameters", "Debug"}(tab)
  in  "device names":refnum<k15>="192.168.1.5"
  in  "IQ rate":dbl=200000.0 format="%#_6p"
  in  "gain":dbl=10.0 format="%#_6f"
  in  "carrier frequency":dbl=2400000000.0 format="%#_6p"
  out "coerced IQ rate":dbl=100000.0 format="%#_6p"
  in  "active antenna":string="TX1"
  in  "error in (no error)":errorcluster
  out "error out":errorcluster
  # "OFDM Transmitter"
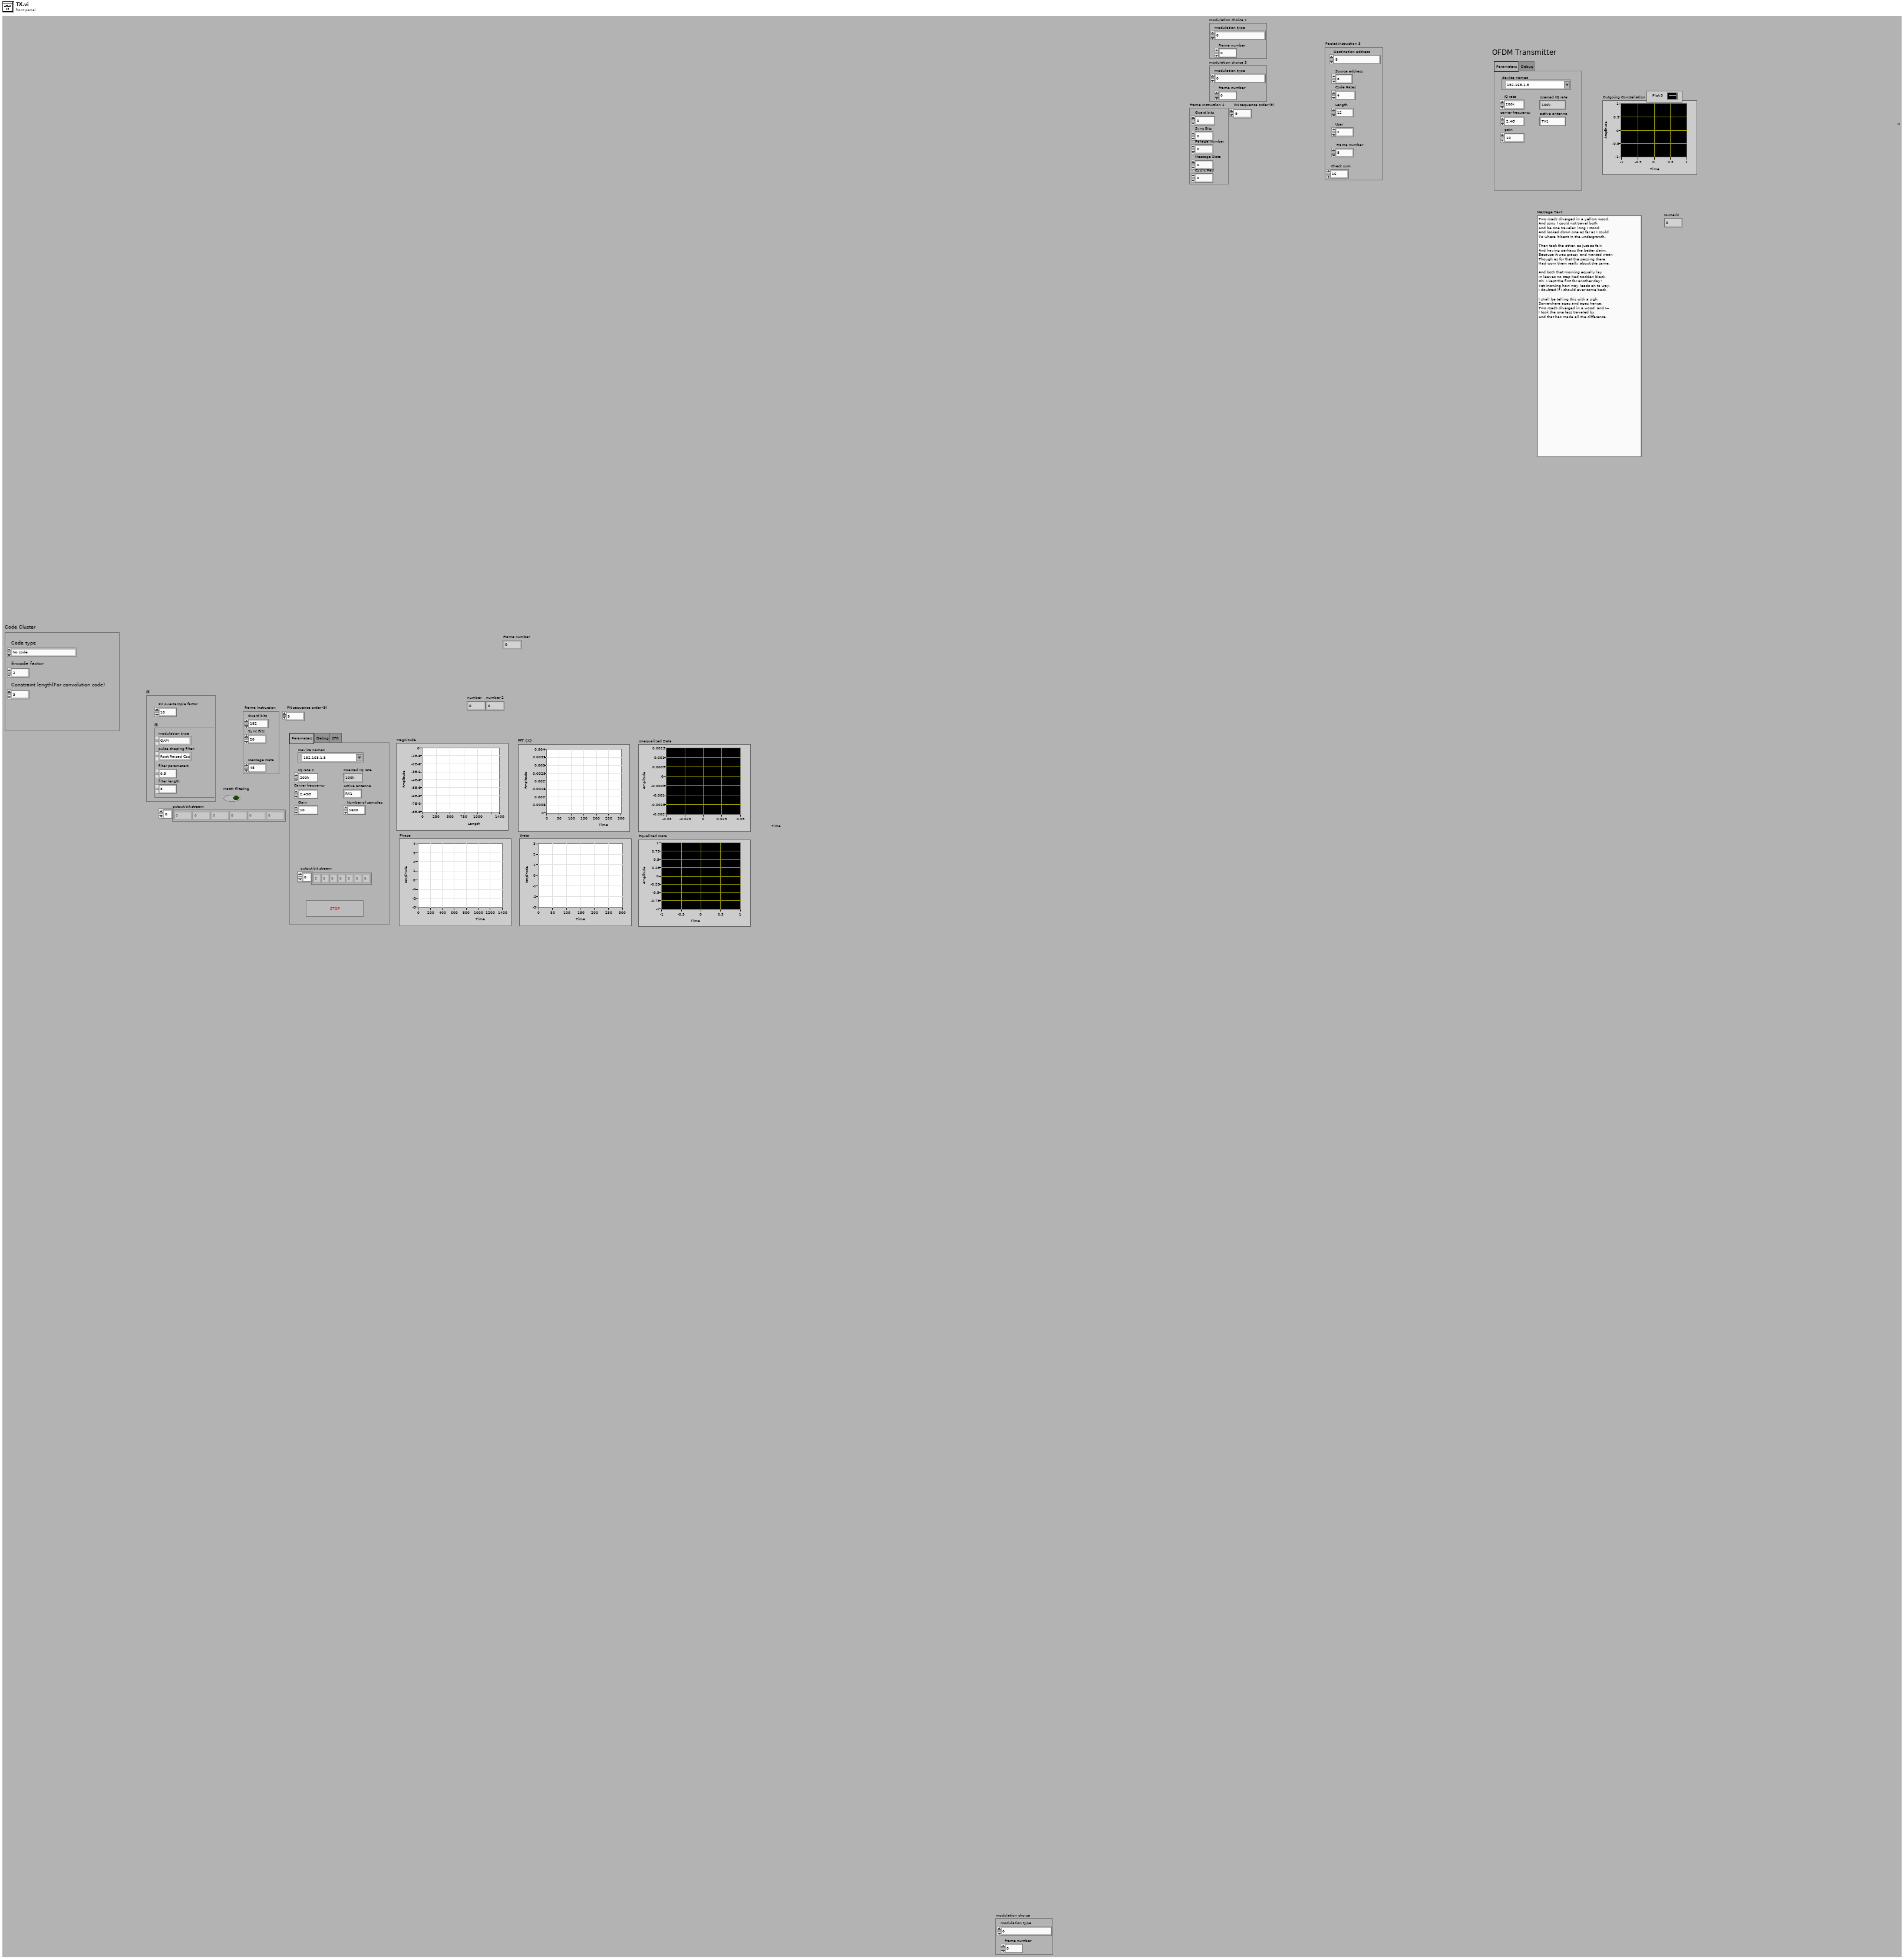
[diagram p1: front panel]
types:
  T1 = cluster{"Guard bits":dbl, "Sync Bits":dbl, "Pakage number":dbl, "Message Data":dbl, "Cyclic Pad":dbl}
  T2 = cluster{"Code type":enum16{"No code", "Convolution code", "Repetition code"}, "Encode factor":i32, "Constraint length(For convolution code)":i32}
  T3 = cluster{"modulation type":dbl, "Frame number":dbl}
  T4 = cluster{"Guard bits":dbl, "Sync Bits":dbl, "Message Data":dbl}
  T5 = cluster{"RX oversample factor":i32, "簇":cluster{"modulation type":u16, "pulse shaping filter":u16, "filter parameters":dbl, "filter length":i32}}
  T6 = cluster{"Code Rates":dbl, "Length":dbl, "Destination address":dbl, "User":dbl, "Source address ":dbl, " Frame number":dbl, " Check sum":dbl}
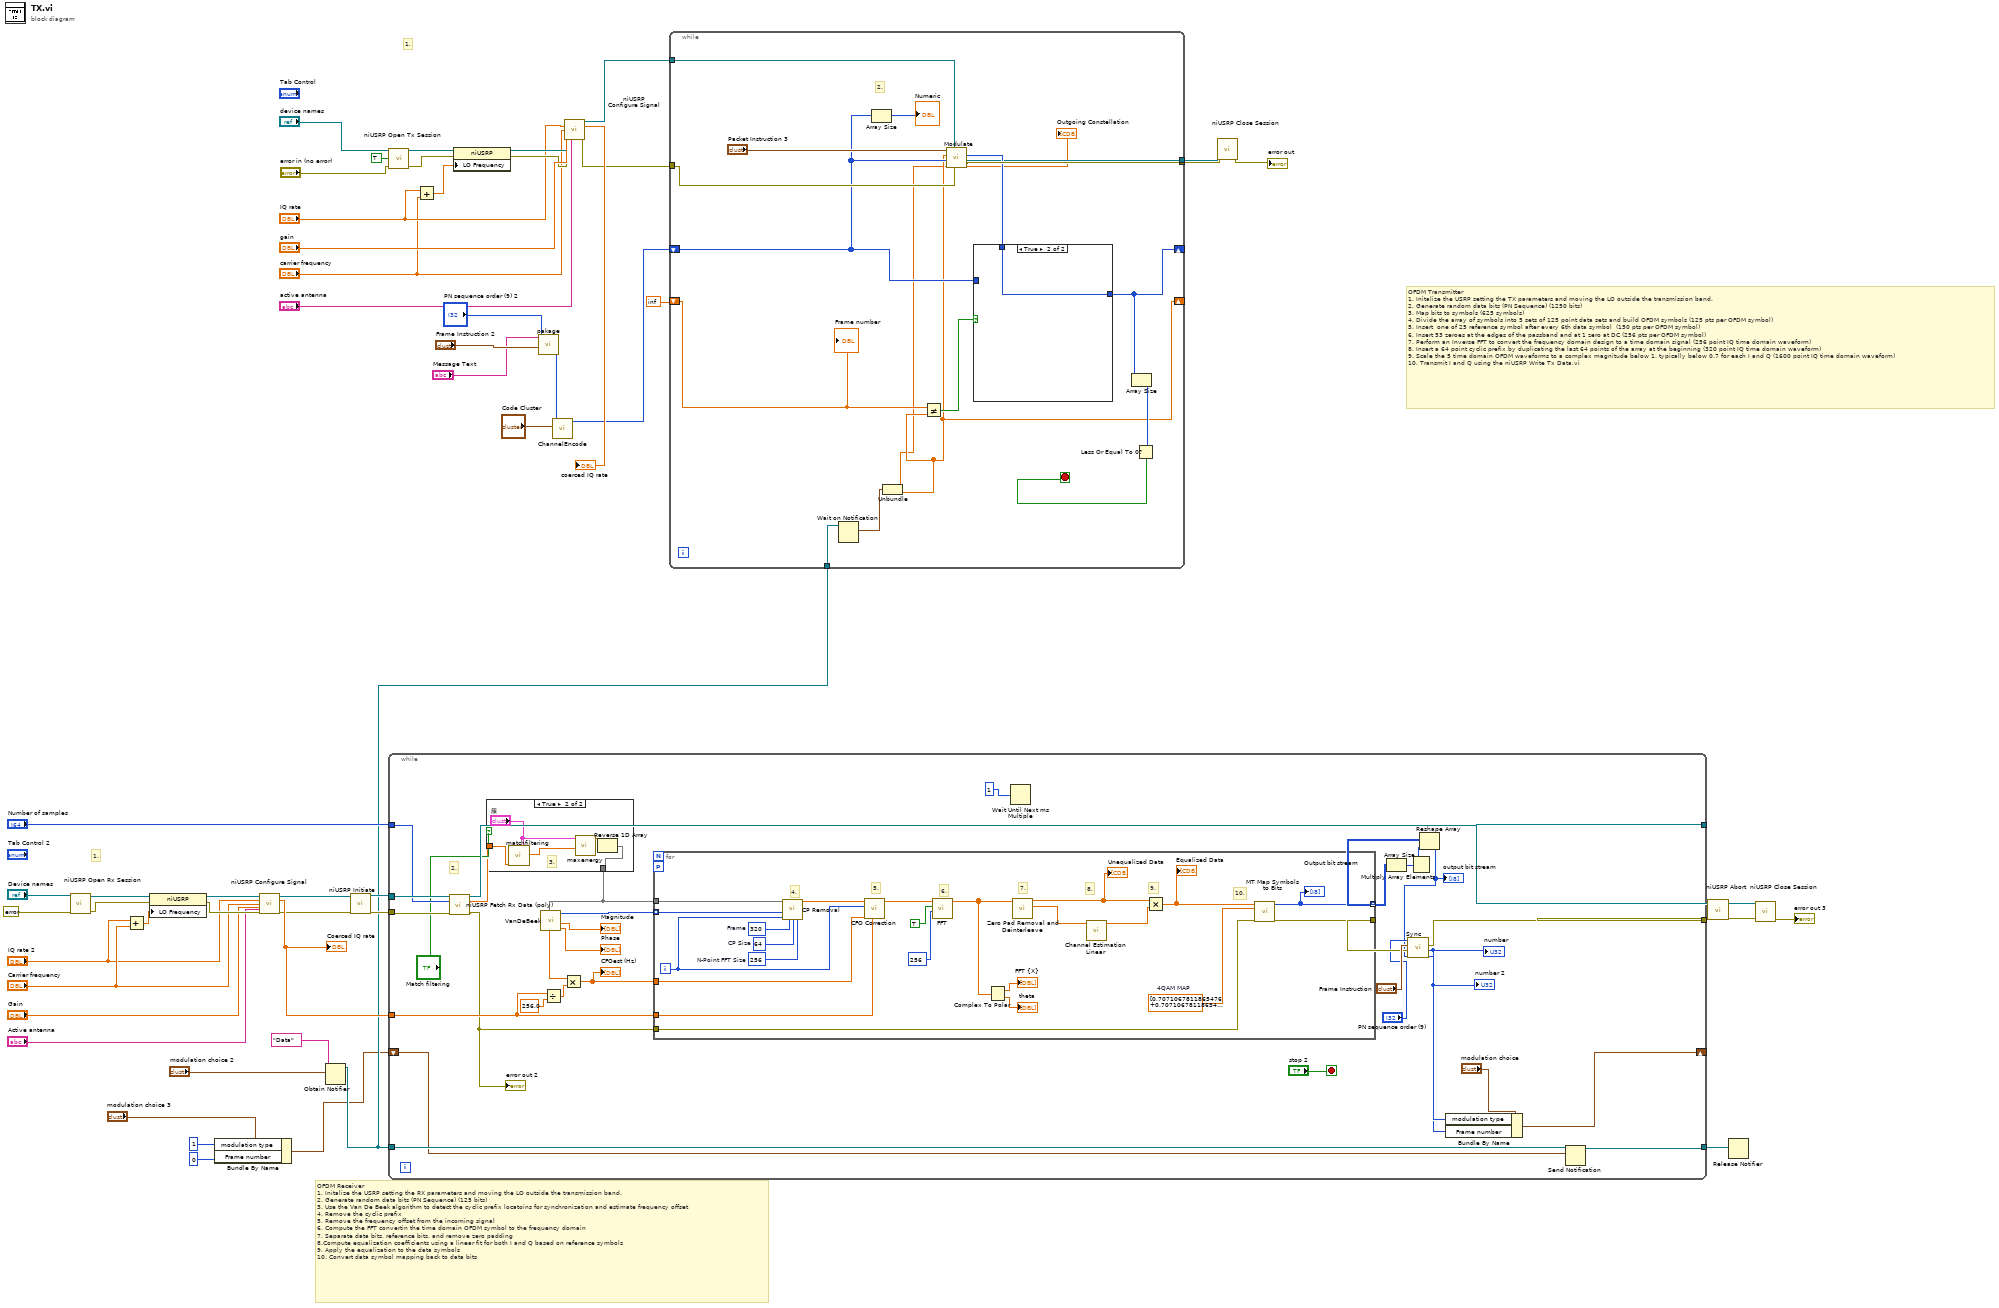
[diagram p0: block diagram]
diagram:
  # "1."
  # "OFDM Receiver\n1. Initalize the USRP setting the RX parameters and moving the LO outside the transmission band.\n2. Generate random data bits (PN Sequence) (125 bits)\n3. Use the Van De Beek algorithm to detect the cyclic prefix locatoins for synchronization and estimate frequency offset\n4. Remove the cyclic prefix\n5. Remove the frequency offset from the incoming signal\n6. Compute the FFT convertin the time domain OFDM symbol to the frequency domain\n7. Separate data bits, reference bits, and remove zero padding\n8.Compute equalization coefficients using a linear fit for both I and Q based on reference symbols \n9. Apply the equalization to the data symbols\n10. Convert data symbol mapping back to data bits"
  # "OFDM Transmitter\n1. Initalize the USRP setting the TX parameters and moving the LO outside the transmission band.\n2. Generate random data bits (PN Sequence) (1250 bits)\n3. Map bits to symbols (625 symbols)\n4. Divide the array of symbols into 5 sets of 125 point data sets and build OFDM symbols (125 pts per OFDM symbol)\n5. Insert  one of 25 reference symbol after every 6th data symbol  (150 pts per OFDM symbol)\n6. Insert 53 zeroes at the edges of the passband and at 1 zero at DC (256 pts per OFDM symbol)\n7. Perform an Inverse FFT to convert the frequency domain design to a time domain signal (256 point IQ time domain waveform)\n8. Insert a 64 point cyclic prefix by duplicating the last 64 points of the array at the beginning (320 point IQ time domain waveform)\n9. Scale the 5 time domain OFDM waveforms to a complex magnitude below 1, typically below 0.7 for each I and Q (1600 point IQ time domain waveform)\n10. Transmit I and Q using the niUSRP Write Tx Data.vi"
  # "1."
  n1 = call <instrlib>:"niUSRP Open Rx Session.vi"("device names"="Device names", "error in (no error)"=errorcluster {"status"=FALSE, "code"=0, "source"=""}) -> ("session handle out"=w35:refnum<k15>, "error out"=w33:errorcluster)  [unwired: 12 in]
  n2 = Add(x="IQ rate 2", y="Carrier frequency") -> (x+y=w27:dbl)
  n3 = property class="niUSRP"(reference=w35, error in=w33, "LO Frequency"=w27) -> (reference out=w34:refnum<k15>, error out=w32:errorcluster)
  n4 = Bundle By Name(cluster="modulation choice 3", "modulation type"=1, "Frame number"=0) -> (w7:T3)
  n5 = call <instrlib>:"niUSRP Configure Signal.vi"("session handle"=w34, "IQ rate"="IQ rate 2", "carrier frequency"="Carrier frequency", "gain"="Gain", "error in (no error)"=w32, "active antenna"="Active antenna") -> ("session handle out"=w17:refnum<k15>, "coerced IQ rate"=w18:dbl, "error out"=w16:errorcluster)  [unwired: 5 in, 2 out]
  "Coerced IQ rate" <- w18
  n6 = Obtain Notifier(name (unnamed)="Data", notification data type="modulation choice 2") -> (notifier out=w11:refnum<notifier>)  [unwired: 2 in, 2 out]
  n7 = call <instrlib>:"niUSRP Initiate.vi"("session handle"=w17, "error in (no error)"=w16) -> ("session handle out"=w37:refnum<k15>, "error out"=w36:errorcluster)  [unwired: 12 in]
  n8 = call <instrlib>:"niUSRP Open Tx Session.vi"("device names"="device names", "reset"=TRUE, "error in (no error)"="error in (no error)") -> ("session handle out"=w45:refnum<k15>, "error out"=w46:errorcluster)  [unwired: 11 in]
  n9 = while {
    tunnel: w37 -> [w86]
    tunnel: w36 -> [w82]
    tunnel: [w85] -> w21
    tunnel: "Number of samples" -> [w83]
    tunnel: w18 -> [w87]
    tunnel: [w72] -> w24
    tunnel: w11 -> [w60]
    tunnel: [w59] -> w12
    shift-right: [w58] -> _
    shift-left: w7 -> [w57]
    stop <- "stop 2" stop-if-true
    # "2."
    n10 = call-poly <instrlib>:"niUSRP Fetch Rx Data (poly).vi"("session handle"=w86, "number of samples"=w83, "error in (no error)"=w82) -> ("session handle out"=w85:refnum<k15>, "data"=w65:cdb[], "error out"=w84:errorcluster)  [unwired: 9 in, 1 out]
    "error out 2" <- w84
    n11 = case shown="True" "Match filtering" {
      tunnel: w65 -> [w89 w91]
      tunnel: [w89 w90] -> w64
      frame False {
      }
      frame True {
        # "3."
        n12 = call "matchfiltering.vi"("数组"=w91, "簇"="簇") -> ("X * Y"=w94:cdb[])  [unwired: 9 in]
        n13 = call "maxenergy.vi"("数组"=w94, "parameters"="簇") -> ("output"=w92:cdb[])  [unwired: 9 in]
        n14 = Reverse 1D Array(array=w92) -> (reversed array=w90:cdb[])
      }
    }
    n15 = call "VanDeBeek.vi"("Input"=w64) -> ("Phase"=→"Phase":dbl[], "Magnitude"=→"Magnitude":dbl[], "Indices"=w79:i32[], "CFOest (Hz)"=w78:dbl[])  [unwired: 6 in, 1 out]
    n16 = Divide(x=w87, y=256.0 ("x")) -> (x/y=w80:dbl)
    n17 = Multiply(x=w78, y=w80) -> (x*y=w75:dbl[])
    "CFOest (Hz)" <- w75
    n18 = for {
      tunnel: w75 -> [w109]
      workers-P: _ -> [_]
      tunnel: w87 -> [w108]
      tunnel: w84 -> [w107]
      tunnel: [w106] -> w73
      tunnel: w79 -> [w101] mode=indexing
      tunnel: w64 -> [w104]
      tunnel: [w98] -> w70 mode=indexing
      i -> [w99]
      w100 = 256  # N-Point FFT Size
      w103 = 64  # CP Size
      w111 = cdb[] [0.7071067811865476+0.7071067811865476i, 0.7071067811865476-0.7071067811865476i, -0.7071067811865476+0.7071067811865476i, -0.7071067811865476-0.7071067811865476i]  # 4QAM MAP
      w102 = 320  # Frame
      # "10."
      # "9."
      # "8."
      # "7."
      # "6."
      # "5."
      # "4."
      n19 = call "CP Removal.vi"("Input"=w104, "Indicies"=w101, "i"=w99, "Frame Size"=w102, "CP Size"=w103, "N-Point FFT Size"=w100) -> ("Output Without CP"=w105:cdb[])  [unwired: 9 in]
      n20 = call "CFO Correction.vi"("fs"=w108, "CFOest (freq)"=w109, "Index"=w99, "Input"=w105) -> ("Output"=w112:cdb[])  [unwired: 7 in]
      n21 = call-poly <vilib>:"FFT.vi"("FFT size"=256, "shift?"=TRUE, "X"=w112) -> ("FFT {X}"=w113:cdb[])  [unwired: 7 in, 1 out]
      n22 = Complex To Polar(r * e^(i*theta)=w113) -> (r=→"FFT {X}":dbl[], theta=→"theta":dbl[])
      n23 = call "Zero Pad Removal and Deinterleave.vi"("Input"=w113) -> ("Ref"=w97:cdb[], "Data"=w95:cdb[])  [unwired: 8 in, 1 out]
      "Unequalized Data" <- w95
      n24 = call "Channel Estimation Linear.vi"("Ref"=w97) -> ("Hest"=w96:cdb[])  [unwired: 9 in, 1 out]
      n25 = Multiply(x=w95, y=w96) -> (x*y=w110:cdb[])
      "Equalized Data" <- w110
      n26 = call-poly <vilib>:"MT Map Symbols to Bits.vi"("symbols"=w110, "symbol map"=w111, "error in (no error)"=w107) -> ("output bit stream"=w98:i8[], "error out"=w106:errorcluster)  [unwired: 11 in]
      "Output bit stream" <- w98
    }
    n27 = Wait Until Next ms Multiple(millisecond multiple=1) -> ()  [unwired: 1 out]
    n28 = Array Size(array=w70) -> (size(s)=w69:i32[])
    n29 = Multiply Array Elements(1:w69) -> (0:w68:i32)
    n30 = Reshape Array(w70, w68) -> (w67:i8[])
    "output bit stream" <- w67
    n31 = call "Sync.vi"("Input Stream"=w67, "error in (no error)"=w73, "Frame Instruction"="Frame Instruction", "PN sequence order (9)"="PN sequence order (9)") -> ("number 2"=w63:u32, "number"=w62:u32, "error out"=w72:errorcluster)  [unwired: 5 in]
    "number" <- w62
    "number 2" <- w63
    n32 = Bundle By Name(cluster="modulation choice", "modulation type"=w63, "Frame number"=w62) -> (w58:T3)
    n33 = Send Notification(notification=w57, notifier=w60) -> (notifier out=w59:refnum<notifier>)  [unwired: 1 in, 1 out]
  }
  n34 = Add(x="IQ rate", y="carrier frequency") -> (x+y=w40:dbl)
  n35 = property class="niUSRP"(reference=w45, error in=w46, "LO Frequency"=w40) -> (reference out=w48:refnum<k15>, error out=w47:errorcluster)
  n36 = call "pakage.vi"("Frame Instruction"="Frame Instruction 2", "PN sequence order (9)"="PN sequence order (9) 2", "text"="Message Text") -> ("appended array"=w2:i8[])  [unwired: 7 in, 1 out]
  n37 = call "ChannelEncode.vi"("Code Cluster"="Code Cluster", "Uncode bits"=w2) -> ("Encoded bits"=w6:i8[])  [unwired: 8 in, 1 out]
  n38 = call <instrlib>:"niUSRP Configure Signal.vi"("session handle"=w48, "IQ rate"="IQ rate", "carrier frequency"="carrier frequency", "gain"="gain", "error in (no error)"=w47, "active antenna"="active antenna") -> ("session handle out"=w44:refnum<k15>, "coerced IQ rate"=→"coerced IQ rate":dbl, "error out"=w39:errorcluster)  [unwired: 5 in, 2 out]
  n39 = while {
    tunnel: w44 -> [w133]
    tunnel: [w134] -> w54
    tunnel: w39 -> [w131]
    shift-right: [w125] -> _
    shift-left: w6 -> [w127]
    shift-right: [w119] -> _
    shift-left: inf -> [w129]
    tunnel: [w126] -> w15
    tunnel: w11 -> [w121]
    stop <- w123 stop-if-true
    # "2."
    n40 = Wait on Notification(notifier=w121) -> (notification=w120:T3)  [unwired: 3 in, 3 out]
    n41 = Array Size(array=w127) -> (size(s)=→"Numeric":i32)
    n42 = Unbundle(w120) -> ("modulation type"=w118:dbl, "Frame number"=w119:dbl)
    n43 = Not Equal?(x=w129, y=w119) -> (x != y?=w128:bool)
    n44 = call "Modulate.vi"("error in (no error)"=w131, "session handle"=w133, "Frame number"=w118, "input bit stream"=w127, "modulation type"=w119, "Frame Instruction 3"="Packet Instruction 3") -> ("Outgoing Constellation"=→"Outgoing Constellation":cdb[], "session handle out"=w126:refnum<k15>, "output bit stream 2"=w130:i32[], "error out"=w134:errorcluster)  [unwired: 2 in]
    n45 = case shown="True" w128 {
      tunnel: [w136 w137] -> w125
      tunnel: w130 -> [_ w137]
      tunnel: w127 -> [w136 _]
      frame False {
      }
      frame True {
      }
    }
    n46 = Array Size(array=w125) -> (size(s)=w124:i32)
    n47 = Less Or Equal To 0?(x=w124) -> (x <= 0?=w123:bool)
    "Frame number" <- w129
  }
  n48 = call <instrlib>:"niUSRP Close Session.vi"("session handle"=w15, "error in (no error)"=w54) -> ("error out"=→"error out":errorcluster)  [unwired: 13 in]
  n49 = call <instrlib>:"niUSRP Abort.vi"("session handle"=w21, "error in (no error)"=w24) -> ("session handle out"=w22:refnum<k15>, "error out"=w23:errorcluster)  [unwired: 12 in]
  n50 = Release Notifier(notifier=w12) -> ()  [unwired: 2 in, 3 out]
  n51 = call <instrlib>:"niUSRP Close Session.vi"("session handle"=w22, "error in (no error)"=w23) -> ("error out"=→"error out 3":errorcluster)  [unwired: 13 in]
